vi "SpikeCurrentCheck.vi"   [LabVIEW 2014]
types:
  T1 = typedef "WPI_MotorControlDeviceRef.ctl" = cluster{"DeviceStatus":errorcluster, "Type":T2, "PWM":cluster{"Controller":T3, "PWM Channel":T4, "DeadBand":T5}, "CAN":cluster{"Device Number":u8, "Control Mode":T6, "Semaphore":T7, "Max Vout":dbl, "TalonSRX Control Mode":T8}, "Invert":bool, "TransformRef":T9, "InvTransformRef":T9}
  T2 = typedef "WPI_MotorControlType.ctl" = enum16{"PWM", "CAN", "CANTalonSRX"}
  T3 = typedef "FPGA_TypedefDigitalModule.ctl" = enum16{"Controller 1"}
  T4 = typedef "FPGA_DIOPWMChannel.ctl" = enum8{"PWM 0", "PWM 1", "PWM 2", "PWM 3", "PWM 4", "PWM 5", "PWM 6", "PWM 7", "PWM 8", "PWM 9", "PWM MXP 0", "PWM MXP 1", "PWM MXP 2", "PWM MXP 3", "PWM MXP 4", "PWM MXP 5", "PWM MXP 6", "PWM MXP 7", "PWM MXP 8", "PWM MXP 9", "Invalid"}
  T5 = typedef "WPI_PWMDeadband.ctl" = cluster{"Name":string, "maxPositivePwm":i32, "minPositivePwm":i32, "centerPwm":i32, "maxNegativePwm":i32, "minNegativePwm":i32, "angularRange":u16}
  T6 = typedef "WPI_CANJaguar_ControlMode.ctl" = enum8{"Percent VBus", "Current", "Speed", "Position", "Voltage"}
  T7 = typedef "Semaphore RefNum" = refnum<k1>
  T8 = typedef "WPI_CANTalonSRX_APIControlMode.ctl" = enum8{"Percent VBus", "Speed", "Position", "Slave", "Unchanged / Invalid"}
  T9 = typedef "WPI_PWMTransform_ConPane.ctl" = refnum<vi>
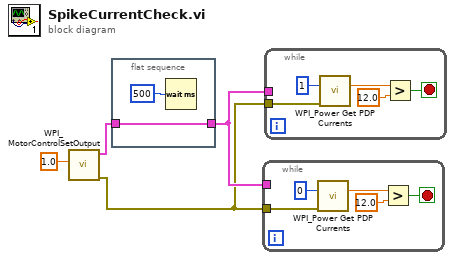
[diagram p0: block diagram]
diagram:
  n1 = call <vilib>:"WPI_MotorControlSetOutput.vi"("Output"=1.0) -> ("error out"=w1:errorcluster, "MotorControlDevRef"=w3:T1)  [unwired: 8 in, 1 out]
  n2 = flat-sequence {
    tunnel: w3 -> [w5]
    tunnel: [w5] -> w2
    frame #0 {
      n3 = Wait (ms)(milliseconds to wait=u32 500) -> ()  [unwired: 1 out]
    }
  }
  n4 = while {
    tunnel: w2 -> [_]
    tunnel: w1 -> [w7]
    stop <- w10 stop-if-true
    n5 = call <vilib>:"WPI_Power Get PDP Currents.vi"("PDP Channel"=0, "error in"=w7) -> ("current (A)"=w9:dbl)  [unwired: 11 in, 2 out]
    n6 = Greater?(x=w9, y=12.0) -> (0:w10:bool)
  }
  n7 = while {
    tunnel: w2 -> [_]
    tunnel: w1 -> [w12]
    stop <- w15 stop-if-true
    n8 = call <vilib>:"WPI_Power Get PDP Currents.vi"("PDP Channel"=1, "error in"=w12) -> ("current (A)"=w14:dbl)  [unwired: 11 in, 2 out]
    n9 = Greater?(x=w14, y=12.0) -> (0:w15:bool)
  }
